vi "Get Timing.vi"(8 "error in (no error)":errorcluster, 11 "General Hardware in":refnum<class "General Hardware.lvclass">) -> (0 "error out":errorcluster, 1 "time delay (ms)":dbl, 2 "frequency (Hz)":dbl, 3 "General Hardware out":refnum<class "General Hardware.lvclass">)   [LabVIEW 2020, in "General Hardware.lvclass"]
uses:
  General Hardware.lvclass
  General Hardware.lvclass/General Hardware.ctl
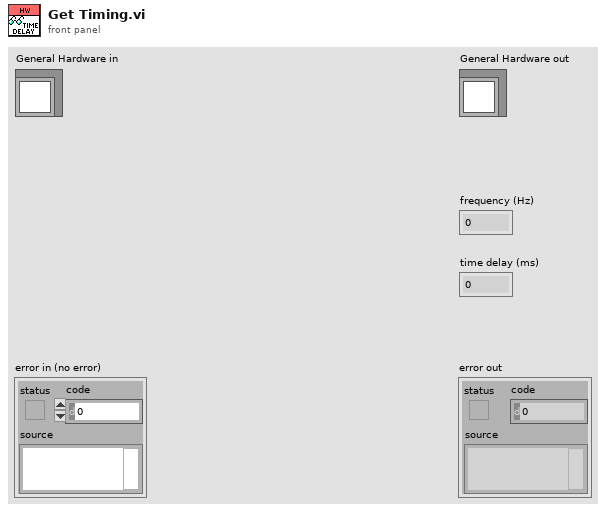
[diagram p1: front panel]
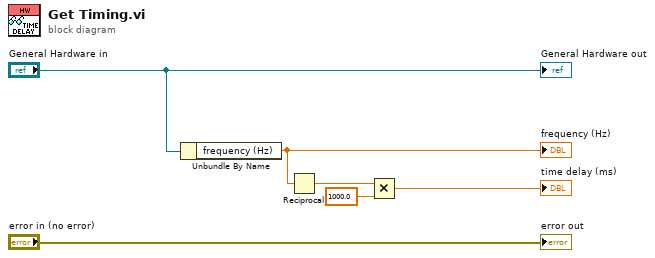
[diagram p0: block diagram]
diagram:
  n1 = Unbundle By Name("General Hardware in") -> ("frequency (Hz)"=w3:dbl)
  "frequency (Hz)" <- w3
  n2 = Reciprocal(x=w3) -> (1/x=w2:dbl)
  n3 = Multiply(x=w2, y=1000.0) -> (x*y=→"time delay (ms)":dbl)
  "error out" <- "error in (no error)"
  "General Hardware out" <- "General Hardware in"
